vi "KINECTGestureProcessing.vi"(0 "Z Wrist Right in":dbl, 1 "Z Wrist Left in":dbl, 2 "Arm Drive in Max (Forward)":dbl, 3 "Arm Drive in Min (Reverse)":dbl) -> (5 "Joystick Data":T1, 6 "Z Wrist Right out":dbl, 7 "Z Wrist Left out":dbl)   [LabVIEW 2011]
doc: "This VI imlements the framework and scheduler for your robotics program. It should not be necessary to modify the framework. You are expected to add your code to the VIs called from Robot Main, the ones located in the Team Code within the project."
uses:
  <vilib>/addons/Kinect/SkeletonVertexTrackState.ctl
  <vilib>/addons/Kinect/Skeleton Vertex Index.ctl
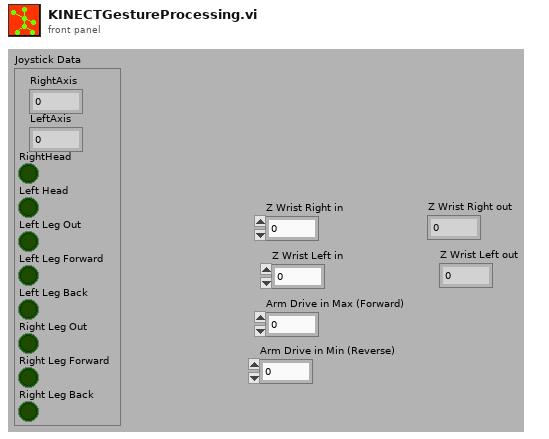
[diagram p1: front panel]
types:
  T1 = cluster{"RightAxis":dbl, "LeftAxis":dbl, "RightHead":bool, "Left Head":bool, "Left Leg Out":bool, "Left Leg Forward":bool, "Left Leg Back":bool, "Right Leg Out":bool, "Right Leg Forward":bool, "Right Leg Back":bool}
  T2 = typedef "Skeleton Vertex Index.ctl" = i32
  T3 = typedef "SkeletonVertexTrackState.ctl" = enum32{"NotTracked", "Inferred", "Tracked"}
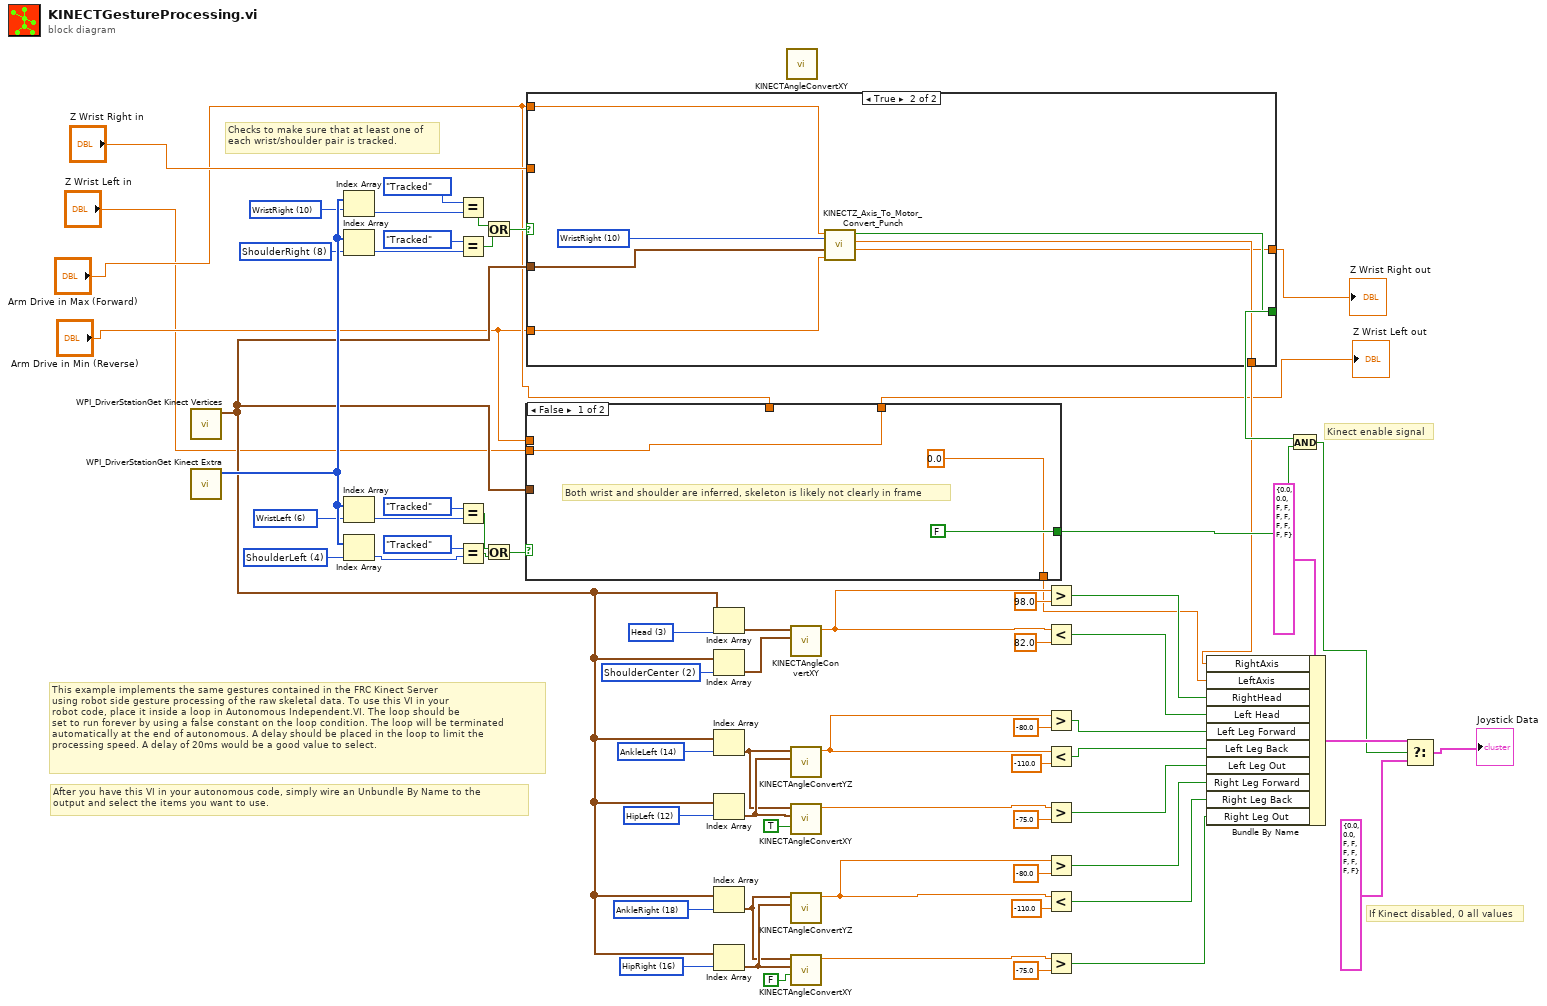
[diagram p0: block diagram]
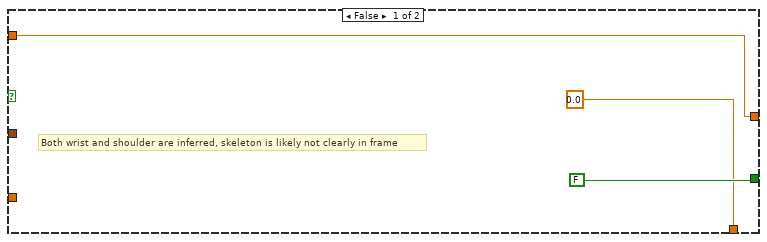
[diagram p2: hidden frame]
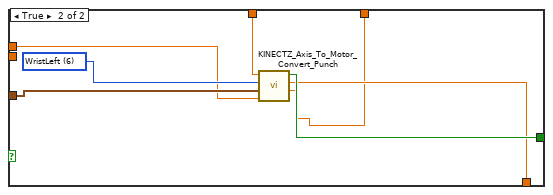
[diagram p3: hidden frame]
diagram:
  w10 = T2 16 items=["HipCenter", "Spine", "ShoulderCenter", "Head", "ShoulderLeft", "ElbowLeft", "WristLeft", "HandLeft", "ShoulderRight", "ElbowRight", "WristRight", "HandRight", "HipLeft", "KneeLeft", "AnkleLeft", "FootLeft", "HipRight", "KneeRight", "AnkleRight", "FootRight"] ("Skeleton Joints")
  w11 = T2 18 items=["HipCenter", "Spine", "ShoulderCenter", "Head", "ShoulderLeft", "ElbowLeft", "WristLeft", "HandLeft", "ShoulderRight", "ElbowRight", "WristRight", "HandRight", "HipLeft", "KneeLeft", "AnkleLeft", "FootLeft", "HipRight", "KneeRight", "AnkleRight", "FootRight"] ("Skeleton Joints")
  w9 = T2 12 items=["HipCenter", "Spine", "ShoulderCenter", "Head", "ShoulderLeft", "ElbowLeft", "WristLeft", "HandLeft", "ShoulderRight", "ElbowRight", "WristRight", "HandRight", "HipLeft", "KneeLeft", "AnkleLeft", "FootLeft", "HipRight", "KneeRight", "AnkleRight", "FootRight"] ("Skeleton Joints")
  w12 = T2 14 items=["HipCenter", "Spine", "ShoulderCenter", "Head", "ShoulderLeft", "ElbowLeft", "WristLeft", "HandLeft", "ShoulderRight", "ElbowRight", "WristRight", "HandRight", "HipLeft", "KneeLeft", "AnkleLeft", "FootLeft", "HipRight", "KneeRight", "AnkleRight", "FootRight"] ("Skeleton Joints")
  w13 = T2 2 items=["HipCenter", "Spine", "ShoulderCenter", "Head", "ShoulderLeft", "ElbowLeft", "WristLeft", "HandLeft", "ShoulderRight", "ElbowRight", "WristRight", "HandRight", "HipLeft", "KneeLeft", "AnkleLeft", "FootLeft", "HipRight", "KneeRight", "AnkleRight", "FootRight"] ("Skeleton Joints")
  w14 = T2 3 items=["HipCenter", "Spine", "ShoulderCenter", "Head", "ShoulderLeft", "ElbowLeft", "WristLeft", "HandLeft", "ShoulderRight", "ElbowRight", "WristRight", "HandRight", "HipLeft", "KneeLeft", "AnkleLeft", "FootLeft", "HipRight", "KneeRight", "AnkleRight", "FootRight"] ("Skeleton Joints")
  w16 = T2 4 items=["HipCenter", "Spine", "ShoulderCenter", "Head", "ShoulderLeft", "ElbowLeft", "WristLeft", "HandLeft", "ShoulderRight", "ElbowRight", "WristRight", "HandRight", "HipLeft", "KneeLeft", "AnkleLeft", "FootLeft", "HipRight", "KneeRight", "AnkleRight", "FootRight"] ("Skeleton Joints")
  w18 = T2 6 items=["HipCenter", "Spine", "ShoulderCenter", "Head", "ShoulderLeft", "ElbowLeft", "WristLeft", "HandLeft", "ShoulderRight", "ElbowRight", "WristRight", "HandRight", "HipLeft", "KneeLeft", "AnkleLeft", "FootLeft", "HipRight", "KneeRight", "AnkleRight", "FootRight"] ("Skeleton Joints")
  w17 = T2 8 items=["HipCenter", "Spine", "ShoulderCenter", "Head", "ShoulderLeft", "ElbowLeft", "WristLeft", "HandLeft", "ShoulderRight", "ElbowRight", "WristRight", "HandRight", "HipLeft", "KneeLeft", "AnkleLeft", "FootLeft", "HipRight", "KneeRight", "AnkleRight", "FootRight"] ("Skeleton Joints")
  w19 = T2 10 items=["HipCenter", "Spine", "ShoulderCenter", "Head", "ShoulderLeft", "ElbowLeft", "WristLeft", "HandLeft", "ShoulderRight", "ElbowRight", "WristRight", "HandRight", "HipLeft", "KneeLeft", "AnkleLeft", "FootLeft", "HipRight", "KneeRight", "AnkleRight", "FootRight"] ("Skeleton Joints")
  # "After you have this VI in your autonomous code, simply wire an Unbundle By Name to the\noutput and select the items you want to use."
  # "This example implements the same gestures contained in the FRC Kinect Server\nusing robot side gesture processing of the raw skeletal data. To use this VI in your\nrobot code, place it inside a loop in Autonomous Independent.VI. The loop should be\nset to run forever by using a false constant on the loop condition. The loop will be terminated\nautomatically at the end of autonomous. A delay should be placed in the loop to limit the \nprocessing speed. A delay of 20ms would be a good value to select."
  # "Checks to make sure that at least one of\neach wrist/shoulder pair is tracked."
  # "If Kinect disabled, 0 all values"
  # "Kinect enable signal"
  n1 = call <vilib>:"WPI_DriverStationGet Kinect Vertices.vi"() -> ("Skeleton Vertices"=w15:cluster{"x":sgl, "y":sgl, "z":sgl}[])  [unwired: 10 in, 1 out]
  n2 = call <vilib>:"WPI_DriverStationGet Kinect Extra.vi"() -> ("Skeleton Tracking State"=w37:T3[])  [unwired: 7 in, 4 out]
  n3 = Index Array(array=w37, index=w19) -> (element=w64:T3)
  n4 = Index Array(array=w37, index=w17) -> (element=w66:T3)
  n5 = Index Array(array=w37, index=w18) -> (element=w58:T3)
  n6 = Index Array(array=w37, index=w16) -> (element=w60:T3)
  n7 = Equal?(x=SkeletonVertexTrackState."Tracked", y=w64) -> (x = y?=w68:bool)
  n8 = Equal?(x=SkeletonVertexTrackState."Tracked", y=w66) -> (x = y?=w67:bool)
  n9 = Equal?(x=SkeletonVertexTrackState."Tracked", y=w58) -> (x = y?=w61:bool)
  n10 = Equal?(x=SkeletonVertexTrackState."Tracked", y=w60) -> (x = y?=w70:bool)
  n11 = Or(x=w68, y=w67) -> (x .or. y?=w69:bool)
  n12 = Or(x=w61, y=w70) -> (x .or. y?=w62:bool)
  n13 = case shown="False" w62 {
    tunnel: w15 -> [_ w79]
    tunnel: [FALSE w78] -> w40
    tunnel: [0.0 w77] -> w7
    tunnel: "Arm Drive in Max (Forward)" -> [_ w76]
    tunnel: "Arm Drive in Min (Reverse)" -> [_ w75]
    tunnel: [w71 w74] -> w2
    tunnel: "Z Wrist Left in" -> [w71 _]
    frame False {
      # "Both wrist and shoulder are inferred, skeleton is likely not clearly in frame"
    }
    frame True {
      w80 = T2 6 items=["HipCenter", "Spine", "ShoulderCenter", "Head", "ShoulderLeft", "ElbowLeft", "WristLeft", "HandLeft", "ShoulderRight", "ElbowRight", "WristRight", "HandRight", "HipLeft", "KneeLeft", "AnkleLeft", "FootLeft", "HipRight", "KneeRight", "AnkleRight", "FootRight"] ("Skeleton Joints")
      n14 = call "KINECTZ_Axis_To_Motor_Convert_Punch.vi"("Arm Drive Min (Reverse)"=w75, "Skeleton Vertices"=w79, "Wrist Input"=w80, "Arm Drive Max (Forward)"=w76) -> ("Z Axis Out"=w74:sgl, "Punch Output (-1 to 1)"=w77:dbl, "In Range ?"=w78:bool)  [unwired: 5 in]
    }
  }
  "Z Wrist Left out" <- w2
  n15 = case shown="True" w69 {
    tunnel: w15 -> [_ w90]
    tunnel: [FALSE w88] -> w41
    tunnel: [0.0 w87] -> w8
    tunnel: "Arm Drive in Max (Forward)" -> [_ w86]
    tunnel: "Arm Drive in Min (Reverse)" -> [_ w85]
    tunnel: [w81 w84] -> w6
    tunnel: "Z Wrist Right in" -> [w81 _]
    frame False {
      # "Both wrist and shoulder are inferred, skeleton is likely not clearly in frame"
    }
    frame True {
      w89 = T2 10 items=["HipCenter", "Spine", "ShoulderCenter", "Head", "ShoulderLeft", "ElbowLeft", "WristLeft", "HandLeft", "ShoulderRight", "ElbowRight", "WristRight", "HandRight", "HipLeft", "KneeLeft", "AnkleLeft", "FootLeft", "HipRight", "KneeRight", "AnkleRight", "FootRight"] ("Skeleton Joints")
      n16 = call "KINECTZ_Axis_To_Motor_Convert_Punch.vi"("Arm Drive Min (Reverse)"=w85, "Skeleton Vertices"=w90, "Wrist Input"=w89, "Arm Drive Max (Forward)"=w86) -> ("Z Axis Out"=w84:sgl, "Punch Output (-1 to 1)"=w87:dbl, "In Range ?"=w88:bool)  [unwired: 5 in]
    }
  }
  "Z Wrist Right out" <- w6
  n17 = Index Array(array=w15, index=w14) -> (element=w36:cluster{"x":sgl, "y":sgl, "z":sgl})
  n18 = Index Array(array=w15, index=w13) -> (element=w35:cluster{"x":sgl, "y":sgl, "z":sgl})
  n19 = Index Array(array=w15, index=w12) -> (element=w31:cluster{"x":sgl, "y":sgl, "z":sgl})
  n20 = Index Array(array=w15, index=w9) -> (element=w32:cluster{"x":sgl, "y":sgl, "z":sgl})
  n21 = Index Array(array=w15, index=w11) -> (element=w33:cluster{"x":sgl, "y":sgl, "z":sgl})
  n22 = Index Array(array=w15, index=w10) -> (element=w34:cluster{"x":sgl, "y":sgl, "z":sgl})
  n23 = call "KINECTAngleConvertXY.vi"() -> ()  [unwired: 10 in, 2 out]
  n24 = call "KINECTAngleConvertXY.vi"("Origin Joint"=w35, "Moving Joint"=w36) -> ("Angle"=w50:dbl)  [unwired: 8 in, 1 out]
  n25 = call "KINECTAngleConvertYZ.vi"("Origin Joint"=w32, "Moving Joint"=w31) -> ("Angle"=w53:dbl)  [unwired: 9 in]
  n26 = call "KINECTAngleConvertXY.vi"("Mirror"=TRUE, "Origin Joint"=w32, "Moving Joint"=w31) -> ("Angle"=w54:dbl)  [unwired: 7 in, 1 out]
  n27 = call "KINECTAngleConvertYZ.vi"("Origin Joint"=w34, "Moving Joint"=w33) -> ("Angle"=w30:dbl)  [unwired: 9 in]
  n28 = call "KINECTAngleConvertXY.vi"("Mirror"=FALSE, "Origin Joint"=w34, "Moving Joint"=w33) -> ("Angle"=w45:dbl)  [unwired: 7 in, 1 out]
  n29 = Greater?(x=w50, y=98.0) -> (0:w43:bool)
  n30 = Less?(x=w50, y=82.0) -> (x < y?=w42:bool)
  n31 = Greater?(x=w53, y=-80.0) -> (0:w28:bool)
  n32 = Less?(x=w53, y=-110.0) -> (x < y?=w27:bool)
  n33 = Greater?(x=w54, y=-75.0) -> (0:w26:bool)
  n34 = Greater?(x=w30, y=-80.0) -> (0:w25:bool)
  n35 = Less?(x=w30, y=-110.0) -> (x < y?=w24:bool)
  n36 = Greater?(x=w45, y=-75.0) -> (0:w23:bool)
  n37 = Bundle By Name(cluster=T1 {"RightAxis"=0.0, "LeftAxis"=0.0, "RightHead"=FALSE, "Left Head"=FALSE, "Left Leg Out"=FALSE, "Left Leg Forward"=FALSE, "Left Leg Back"=FALSE, "Right Leg Out"=FALSE, "Right Leg Forward"=FALSE, "Right Leg Back"=FALSE} ("f"), "RightAxis"=w8, "LeftAxis"=w7, "RightHead"=w43, "Left Head"=w42, "Left Leg Forward"=w28, "Left Leg Back"=w27, "Left Leg Out"=w26, "Right Leg Forward"=w25, "Right Leg Back"=w24, "Right Leg Out"=w23) -> (w39:T1)
  n38 = And(x=w41, y=w40) -> (x .and. y?=w38:bool)
  n39 = Select(t=w39, s=w38, f=T1 {"RightAxis"=0.0, "LeftAxis"=0.0, "RightHead"=FALSE, "Left Head"=FALSE, "Left Leg Out"=FALSE, "Left Leg Forward"=FALSE, "Left Leg Back"=FALSE, "Right Leg Out"=FALSE, "Right Leg Forward"=FALSE, "Right Leg Back"=FALSE}) -> (s? t:f=→"Joystick Data":T1)
